vi "Set Constant Action Data.vi"(8 "error in (no error)":errorcluster, 10 "Constant Action Data":variant, 11 "Virt Instr Base in":refnum<class "Virt Instr Base.lvclass">) -> (0 "error out":errorcluster, 3 "Virt Instr Base out":refnum<class "Virt Instr Base.lvclass">)   [LabVIEW 2023, in "HAL GOOP4.lvlib" / "Virt Instr Base.lvclass"]
uses:
  Virt Instr Base.lvclass
  Virt Instr Base.lvclass/Virt Instr Base.ctl
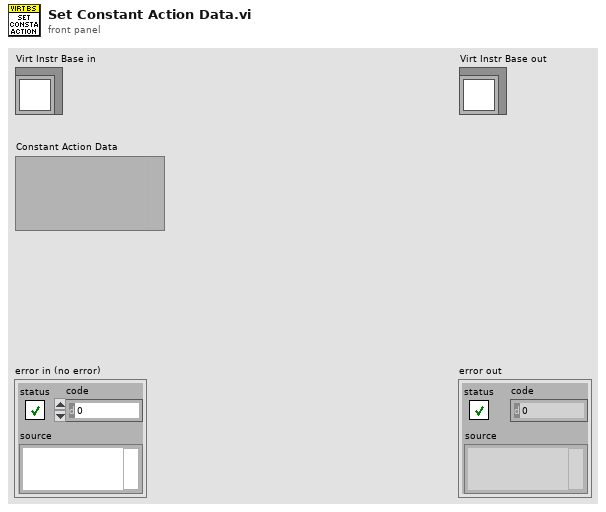
[diagram p1: front panel]
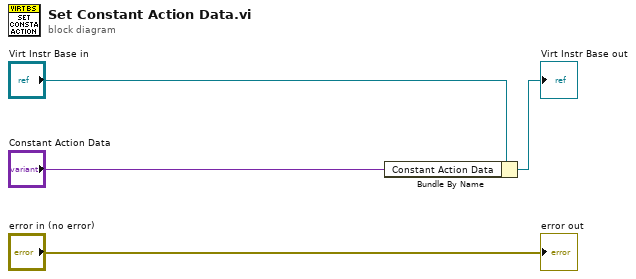
[diagram p0: block diagram]
diagram:
  n1 = Bundle By Name(cluster="Virt Instr Base in", "Constant Action Data"="Constant Action Data") -> (→"Virt Instr Base out":refnum<class "Virt Instr Base.lvclass">)
  "error out" <- "error in (no error)"
